vi "UnsortAndBeep.vi"() -> ()   [LabVIEW 2015]
uses:
  <vilib>/Utility/inputDevices.llb/keyboardAcquire.vi
  <vilib>/Utility/inputDevices.llb/closeKeyboard.vi
panel:
  out "Timer":dbl[](array[numeric])
  in  "stop":bool
  out "Keys Pressed":T1(array[ring])
  out "Sequence":T1(array[ring])
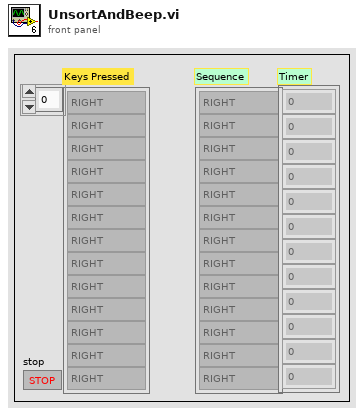
[diagram p1: front panel]
types:
  T1 = enum16{"0", "1", "2", "3", "4", "5", "6", "7", "8", "9", "A", "B", "C", "D", "E", "F", "G", "H", "I", "J", "K", "L", "M", "N", "O", "P", "Q", "R", "S", "T", "U", "V", "W", "X", "Y", "Z", "F1", "F2", "F3", "F4", "F5", "F6", "F7", "F8", "F9", "F10", "F11", "F12", "F13", "F14", "F15", "ADD", "BACK", "BACKSLASH", "CAPITAL", "COMMA", "DECIMAL", "DELETE", "DIVIDE", "DOWN", "END", "EQUALS", "ESCAPE", "GRAVE (`)", "HOME", "INSERT", "LBRACKET", "LCONTROL", "LEFT", "L ALT", "LSHIFT", "LWIN", "MINUS", "MULTIPLY", "NEXT", "NUMLOCK", "NUMPAD_0", "NUMPAD_1", "NUMPAD_2", "NUMPAD_3", "NUMPAD_4", "NUMPAD_5", "NUMPAD_6", "NUMPAD_7", "NUMPAD_8", "NUMPAD_9", "PAUSE", "PERIOD", "PRIOR (PG UP)", "RBRACKET", "RCONTROL", "RETURN", "RIGHT", "R ALT", "RSHIFT", "RWIN", "SCROLL", "SEMICOLON", "SLASH", "SPACE", "SUBTRACT", "TAB", "UP", "ENTER (num pad)", "' (quote)"}[]
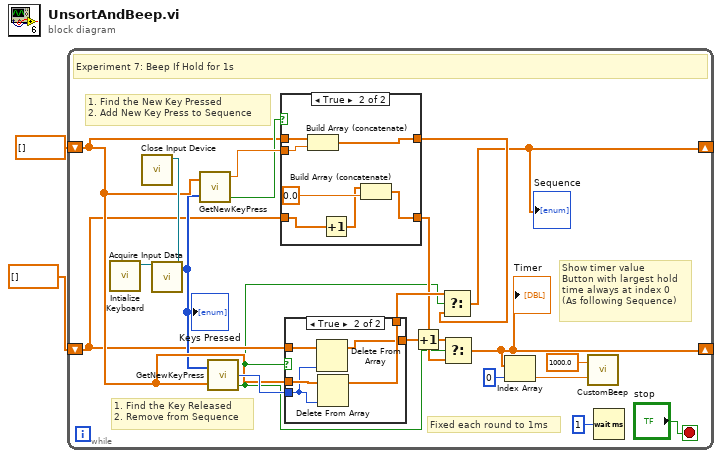
[diagram p0: block diagram]
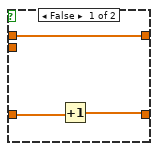
[diagram p3: hidden frame]
diagram:
  n1 = while {
    shift-right: [w9] -> _
    shift-left: dbl[] [] -> [w17]
    shift-right: [w8] -> _
    shift-left: dbl[] [] -> [w11]
    stop <- "stop" stop-if-true
    # "Show timer value\nButton with largest hold\ntime always at index 0\n(As following Sequence)"
    # "Fixed each round to 1ms"
    # "1. Find the Key Released\n2. Remove from Sequence"
    # "1. Find the New Key Pressed\n2. Add New Key Press to Sequence"
    # "Experiment 7: Beep If Hold for 1s"
    n2 = call <vilib>:"Intialize Keyboard.vi"() -> ("device ID"=w22:refnum<k1>)  [unwired: 10 in, 1 out]
    n3 = call-poly <vilib>:"Acquire Input Data.vi"("device ID"=w22) -> ("device ID"=w21:refnum<k1>, "keys pressed"=w14:T1)  [unwired: 16 in, 1 out]
    "Keys Pressed" <- w14
    n4 = call-poly <vilib>:"Close Input Device.vi"("device ID"=w21) -> ()  [unwired: 9 in, 1 out]
    n5 = call "GetNewKeyPress.vi"("n Array"=w17, "n+1 Array"=w14) -> ("Extracted Different"=w20:dbl, "Changes?"=w19:bool)  [unwired: 1 out]
    n6 = call "GetNewKeyPress.vi"("n Array"=w14, "n+1 Array"=w17) -> ("Extracted Index"=w18:i32, "Changes?"=w10:bool)  [unwired: 1 out]
    n7 = case shown="True" w19 {
      tunnel: w20 -> [_ w38]
      tunnel: w17 -> [w33 w40]
      tunnel: [w33 w39] -> w15
      tunnel: w11 -> [w32 w35]
      tunnel: [w31 w37] -> w12
      frame False {
        n8 = Increment(x=w32) -> (x+1=w31:dbl[])
      }
      frame True {
        n9 = Build Array (concatenate)(w40, w38) -> (w39:dbl[])
        n10 = Increment(x=w35) -> (x+1=w34:dbl[])
        n11 = Build Array (concatenate)(w34, 0.0 ("Numeric")) -> (w37:dbl[])
      }
    }
    n12 = case shown="True" w10 {
      tunnel: w18 -> [_ w27]
      tunnel: w17 -> [w25 w30]
      tunnel: [w25 w29] -> w16
      tunnel: w11 -> [w24 w28]
      tunnel: [w24 w26] -> w3
      frame False {
      }
      frame True {
        n13 = Delete From Array(array=w28, index=w27) -> (array with subset deleted=w26:dbl[])  [unwired: 1 in, 1 out]
        n14 = Delete From Array(array=w30, index=w27) -> (array with subset deleted=w29:dbl[])  [unwired: 1 in, 1 out]
      }
    }
    n15 = Increment(x=w3) -> (x+1=w4:dbl[])
    n16 = Select(t=w16, s=w10, f=w15) -> (s? t:f=w9:dbl[])
    "Sequence" <- w9
    n17 = Select(t=w4, s=w10, f=w12) -> (s? t:f=w8:dbl[])
    "Timer" <- w8
    n18 = Index Array(array=w8, index=0) -> (element=w5:dbl)
    n19 = call "CustomBeep.vi"("Holding time"=w5, "Threshold to Beep"=1000.0) -> ()
    n20 = Wait (ms)(milliseconds to wait=u32 1) -> ()  [unwired: 1 out]
  }
